vi "TreeSelectionsToStringArray.vi"(8 "error in (no error)":errorcluster, 11 "Channel Selection":string[](array[string])) -> (0 "error out":errorcluster, 3 "Array":string[][](array[string]))   [LabVIEW 2018]
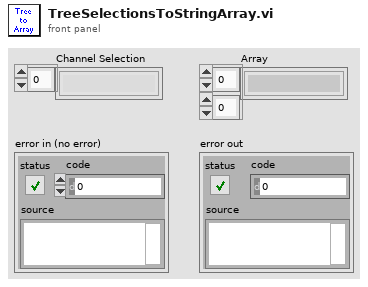
[diagram p1: front panel]
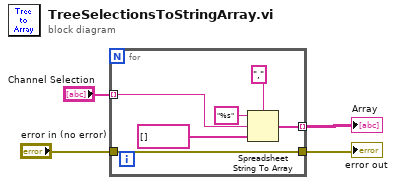
[diagram p0: block diagram]
diagram:
  n1 = for {
    tunnel: "Channel Selection" -> [w10] mode=indexing
    tunnel: [w7] -> w1 mode=indexing
    tunnel: [w5] -> w3
    tunnel: "error in (no error)" -> [w5]
    n2 = Spreadsheet String To Array(delimiter (Tab)=",", format string="%s", spreadsheet string=w10, array type (2D Dbl)=string[] []) -> (array=w7:string[])
  }
  "error out" <- w3
  "Array" <- w1
